vi "Write Sub Panel Coin.vi"(8 "error in (no error)":errorcluster, 10 "Sub Panel Coin":refnum<vi>, 11 "USD Actor in":refnum<class "USD Actor.lvclass">) -> (0 "error out":errorcluster, 3 "USD Actor out":refnum<class "USD Actor.lvclass">)   [LabVIEW 2020, in "USD Actor.lvlib" / "USD Actor.lvclass"]
uses:
  USD Actor.lvclass
  USD Actor.lvclass/USD Actor.ctl
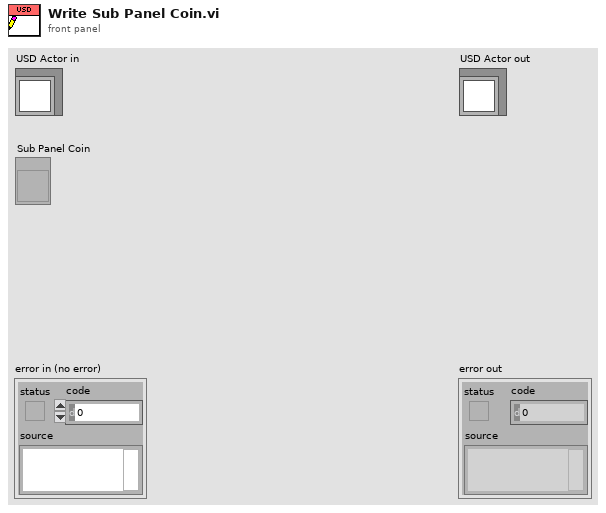
[diagram p1: front panel]
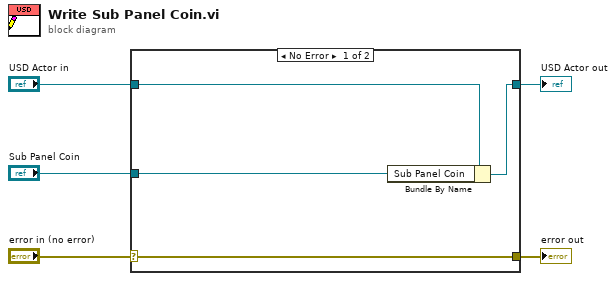
[diagram p0: block diagram]
diagram:
  n1 = case shown="No Error" "error in (no error)" {
    selector: "error in (no error)" -> [w9 w10]
    tunnel: [w9 w10] -> w4
    tunnel: [w7 w11] -> w2
    tunnel: "USD Actor in" -> [w8 w11]
    tunnel: "Sub Panel Coin" -> [w6 _]
    frame No Error {
      n2 = Bundle By Name(cluster=w8, "Sub Panel Coin"=w6) -> (w7:refnum<class "USD Actor.lvclass">)
    }
    frame Error {
    }
  }
  "error out" <- w4
  "USD Actor out" <- w2
